vi "Read Fixture RTD.vi"(0 "error in (no error)":errorcluster, 2 "Measurements (10)":i32=10, 3 "logical name":refnum<k15>="IVI-KE2000") -> (7 "error out":errorcluster, 9 "Temperature StdDev":dbl=nan format="%0.2f", 10 "Mean Temperature (C)":dbl=nan)   [LabVIEW 2010]
doc: "This function performs 4-wire resistance measurements with the 10k ohm range, then changes the meter range to 100M ohms to reduce RTD self-heating."
uses:
  <vilib>/Analysis/NI_AALBase.lvlib
panel:
  out "temperatures":dbl[](array[numeric]) format="%.3f"
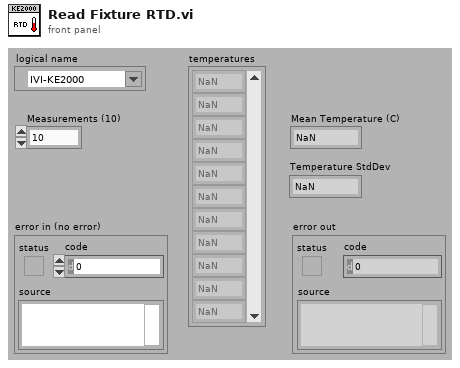
[diagram p1: front panel]
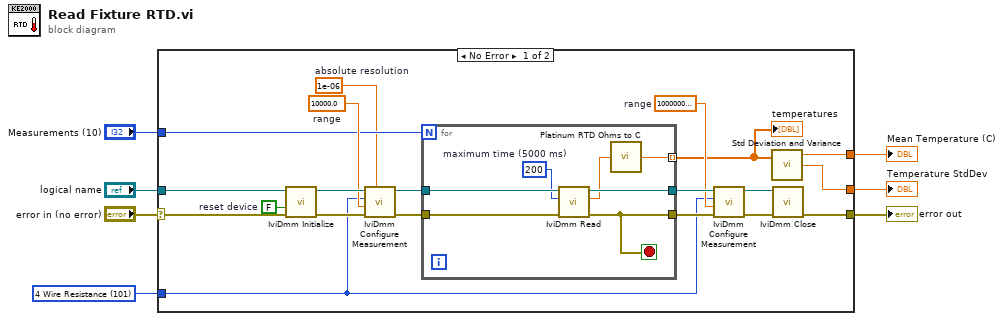
[diagram p0: block diagram]
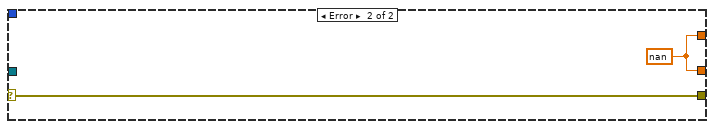
[diagram p2: hidden frame]
diagram:
  w2 = 101 items=["DC Volts"=1, "AC Volts"=2, "DC Current"=3, "AC Current"=4, "2 Wire Resistance"=5, "4 Wire Resistance"=101, "AC + DC Volts"=106, "AC + DC Current"=107, "Frequency"=104, "Period"=105, "Temperature"=108] ("measurement function (DC Volts)")
  n1 = case shown="No Error" "error in (no error)" {
    selector: "error in (no error)" -> [w17 w36]
    tunnel: [w24 w36] -> w7
    tunnel: "Measurements (10)" -> [w21 _]
    tunnel: [w19 w35] -> w5
    tunnel: [w18 w35] -> w4
    tunnel: w2 -> [w9 _]
    tunnel: "logical name" -> [w15 _]
    frame No Error {
      w10 = 100000000.0  # range
      w16 = FALSE  # reset device
      w20 = 1e-06  # absolute resolution
      w26 = 10000.0  # range
      n2 = call <vilib>:"IviDmm Initialize.vi"("error in (no error)"=w17, "reset device (True)"=w16, "logical name (\"SampleDmm\")"=w15) -> ("error out"=w25:errorcluster, "instrument handle out"=w27:refnum<k15>)  [unwired: 7 in]
      n3 = call <vilib>:"IviDmm Configure Measurement.vi"("absolute resolution (0.001)"=w20, "error in (no error)"=w25, "range (-1.0: Auto)"=w26, "measurement function (DC Volts)"=w9, "instrument handle"=w27) -> ("error out"=w22:errorcluster, "instrument handle out"=w23:refnum<k15>)  [unwired: 5 in]
      n4 = for {
        N: w21 -> [_]
        tunnel: w22 -> [w33]
        tunnel: [w32] -> w14
        tunnel: w23 -> [w34]
        tunnel: [w31] -> w11
        tunnel: [w28] -> w8 mode=indexing
        stop <- w32 stop-if-true
        w30 = 200  # maximum time (5000 ms)
        n5 = call <vilib>:"IviDmm Read.vi"("error in (no error)"=w33, "maximum time (5000 ms)"=w30, "instrument handle"=w34) -> ("error out"=w32:errorcluster, "reading"=w29:dbl, "instrument handle out"=w31:refnum<k15>)  [unwired: 6 in]
        n6 = call "Platinum RTD Ohms to C.vi"("Rt"=w29) -> ("Temp (C)"=w28:dbl)
      }
      "temperatures" <- w8
      n7 = call <vilib>:"IviDmm Configure Measurement.vi"("error in (no error)"=w14, "range (-1.0: Auto)"=w10, "measurement function (DC Volts)"=w9, "instrument handle"=w11) -> ("error out"=w13:errorcluster, "instrument handle out"=w12:refnum<k15>)  [unwired: 6 in]
      n8 = call <vilib>:"Std Deviation and Variance.vi"("X"=w8) -> ("mean"=w19:dbl, "standard deviation"=w18:dbl)  [unwired: 1 in, 1 out]
      n9 = call <vilib>:"IviDmm Close.vi"("error in (no error)"=w13, "instrument handle"=w12) -> ("error out"=w24:errorcluster)  [unwired: 9 in]
    }
    frame Error {
      w35 = nan ("standard deviation")
    }
  }
  "error out" <- w7
  "Mean Temperature (C)" <- w5
  "Temperature StdDev" <- w4
